vi "Boiler Controller.vi"(8 "error in":errorcluster, 10 "Notifiers":T1, 11 "Message Queues":T2) -> (0 "error out":errorcluster)   [LabVIEW 2014]
uses:
  support/Message Queue/All Message Queues.ctl
  support/Message Queue/Message Cluster.ctl
  support/Notifiers/Notifiers.ctl
  <vilib>/Utility/error.llb/Error Cluster From Error Code.vi
  <vilib>/ErrorRing/Error Ring.xnode
  support/Message Queue/Message Queue.lvlib
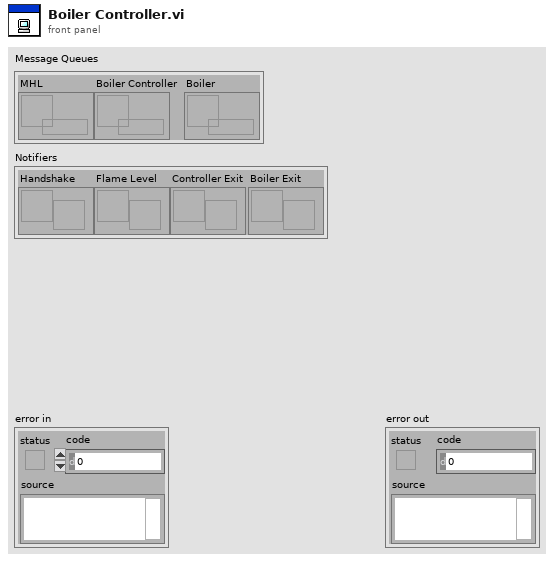
[diagram p1: front panel]
types:
  T1 = typedef "Notifiers.ctl" = cluster{"Handshake":refnum<notifier>, "Flame Level":refnum<notifier>, "Controller Exit":refnum<notifier>, "Boiler Exit":refnum<notifier>}
  T2 = typedef "Message Queue.lvlib/All Message Queues.ctl" = cluster{"MHL":refnum<queue>, "Boiler Controller":refnum<queue>, "Boiler":refnum<queue>}
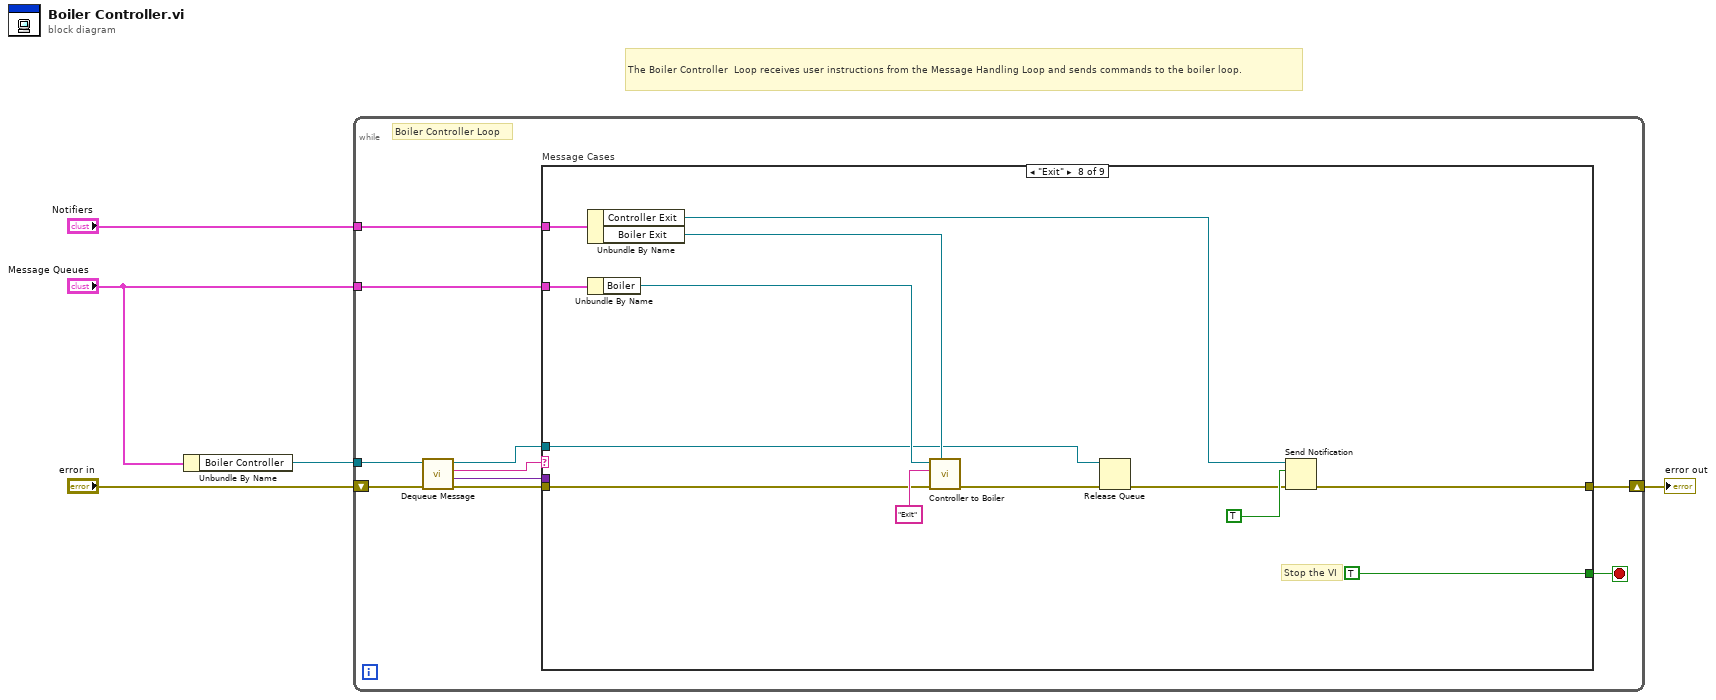
[diagram p0: block diagram]
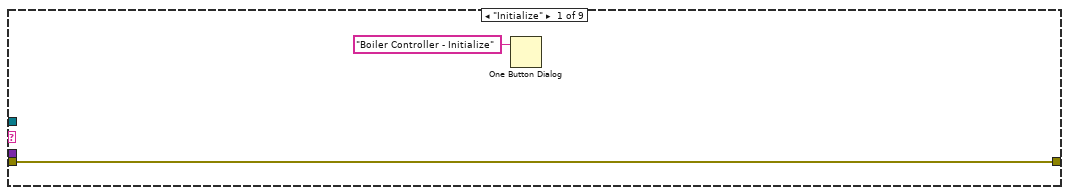
[diagram p2: hidden frame]
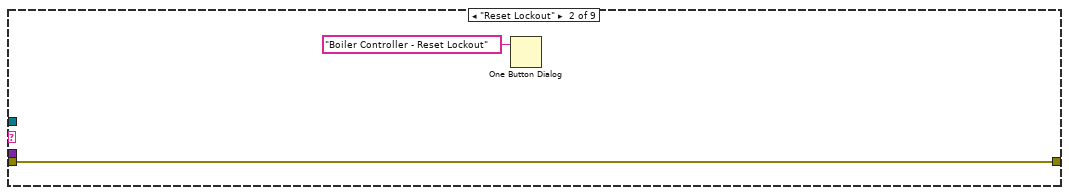
[diagram p3: hidden frame]
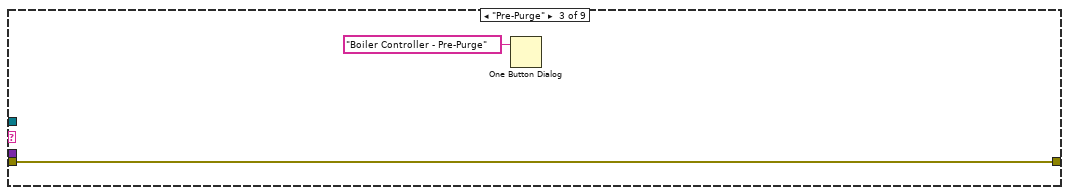
[diagram p4: hidden frame]
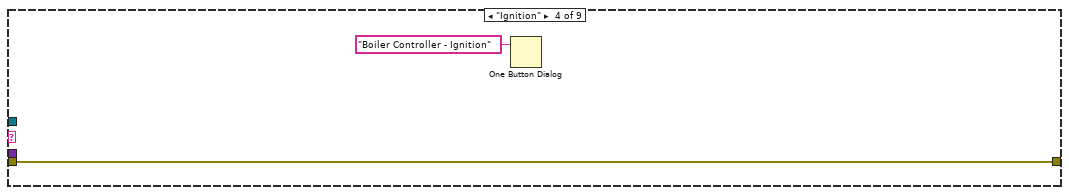
[diagram p5: hidden frame]
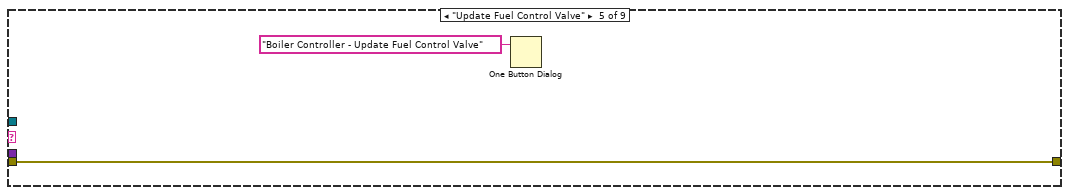
[diagram p6: hidden frame]
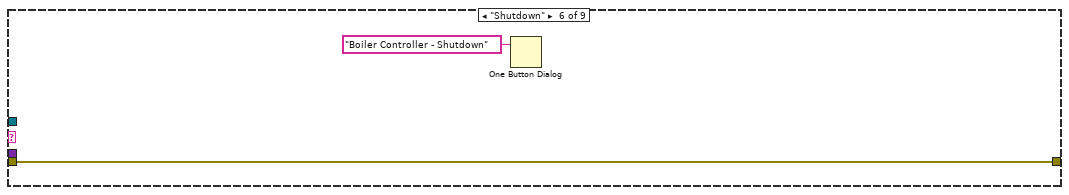
[diagram p7: hidden frame]
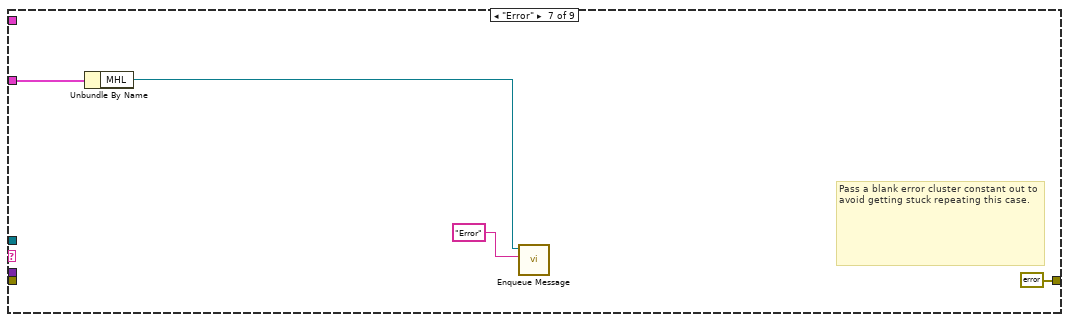
[diagram p8: hidden frame]
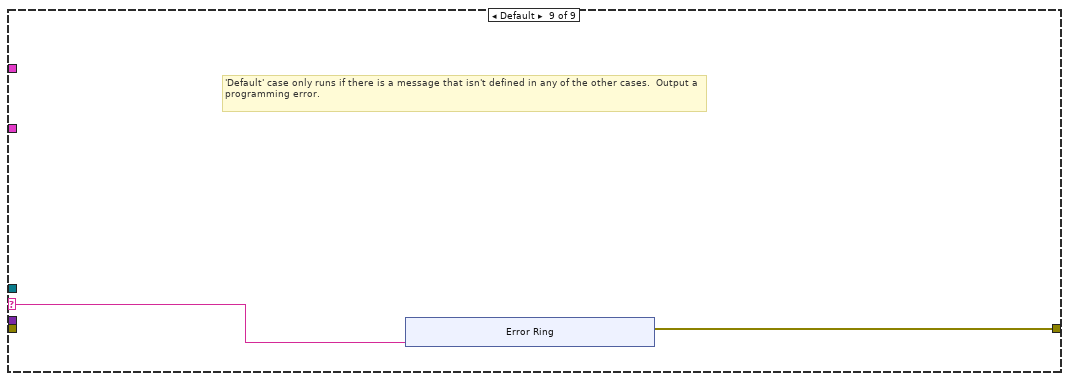
[diagram p9: hidden frame]
diagram:
  # "The Boiler Controller  Loop receives user instructions from the Message Handling Loop and sends commands to the boiler loop."
  n1 = Unbundle By Name("Message Queues") -> ("Boiler Controller"=w3:refnum<queue>)
  n2 = while {
    tunnel: w3 -> [w9]
    shift-right: [w8] -> w5
    shift-left: "error in" -> [w14]
    tunnel: "Message Queues" -> [w7]
    tunnel: "Notifiers" -> [w6]
    stop <- w15 stop-if-true
    # "Boiler Controller Loop"
    n3 = call "Dequeue Message.vi"("error in (no error)"=w14, "Message Queue"=w9) -> ("error out"=w13:errorcluster, "Message Data"=w11:variant, "Message"=w12:string, "dup Message Queue"=w10:refnum<queue>)  [unwired: 6 in]
    n4 = case "Message Cases" shown="\"Exit\"" w12 {
      selector: w12 -> [_ _ _ _ _ _ _ _ w45]
      tunnel: w10 -> [_ _ _ _ _ _ _ w37 _]
      tunnel: w13 -> [w17 w19 w21 w23 w25 w27 _ w36 _]
      tunnel: [w17 w19 w21 w23 w25 w27 errorcluster {"status"=FALSE, "code"=0, "source"=""} ("error out") w34 w46] -> w8
      tunnel: [_ _ _ _ _ _ _ TRUE _] -> w15
      tunnel: w11 -> [_ _ _ _ _ _ _ _ _]
      tunnel: w7 -> [_ _ _ _ _ _ w30 w33 _]
      tunnel: w6 -> [_ _ _ _ _ _ _ w32 _]
      frame "Initialize" {
        n5 = One Button Dialog(message="Boiler Controller - Initialize") -> ()  [unwired: 1 in, 1 out]
      }
      frame "Reset Lockout" {
        n6 = One Button Dialog(message="Boiler Controller - Reset Lockout") -> ()  [unwired: 1 in, 1 out]
      }
      frame "Pre-Purge" {
        n7 = One Button Dialog(message="Boiler Controller - Pre-Purge") -> ()  [unwired: 1 in, 1 out]
      }
      frame "Ignition" {
        n8 = One Button Dialog(message="Boiler Controller - Ignition") -> ()  [unwired: 1 in, 1 out]
      }
      frame "Update Fuel Control Valve" {
        n9 = One Button Dialog(message="Boiler Controller - Update Fuel Control Valve") -> ()  [unwired: 1 in, 1 out]
      }
      frame "Shutdown" {
        n10 = One Button Dialog(message="Boiler Controller - Shutdown") -> ()  [unwired: 1 in, 1 out]
      }
      frame "Error" {
        # "Pass a blank error cluster constant out to avoid getting stuck repeating this case."
        n11 = Unbundle By Name(w30) -> ("MHL"=w29:refnum<queue>)
        n12 = call "Enqueue Message.vi"("Message"="Error", "Message Queue"=w29) -> ()  [unwired: 8 in, 2 out]
      }
      frame "Exit" {
        # "Stop the VI"
        n13 = Unbundle By Name(w32) -> ("Controller Exit"=w39:refnum<notifier>, "Boiler Exit"=w41:refnum<notifier>)
        n14 = Unbundle By Name(w33) -> ("Boiler"=w38:refnum<queue>)
        n15 = call "Controller to Boiler.vi"("Notifier"=w41, "error in"=w36, "Message"="Exit", "Boiler Queue in"=w38) -> ("error out"=w44:errorcluster)  [unwired: 5 in, 2 out]
        n16 = Release Queue(queue=w37, error in (no error)=w44) -> (error out=w40:errorcluster)  [unwired: 1 in, 2 out]
        n17 = Send Notification(notification=TRUE, notifier=w39, error in (no error)=w40) -> (error out=w34:errorcluster)  [unwired: 1 out]
      }
      frame Default {
        # "'Default' case only runs if there is a message that isn't defined in any of the other cases.  Output a programming error."
        n18 = xnode "Error Ring"("parameter 0"=w45) -> ("error out"=w46:errorcluster)
      }
    }
  }
  "error out" <- w5
